vi "ScriptCreateEIO.vi"(8 "direction":T9, 9 "nodes links":string[](array[string]), 10 "Position":cluster{"Left":i32, "Top":i32}, 11 "TopLevelDiagram in":refnum<vi>) -> (0 "terminal names":string[](array[string]), 1 "FPGA I/O out":refnum<vi>, 2 "FPGA I/O in":refnum<vi>, 3 "I/O terminal":refnum<vi>)   [LabVIEW 2014]
uses:
  <vilib>/eio/EIO_TerminalDirection.ctl
  <vilib>/XNodeSupport/XNodeTerm3Array.ctl
  <vilib>/XNodeSupport/XNodeTerm3.ctl
  <vilib>/XNodeSupport/XNodeString.ctl
  <vilib>/XNodeSupport/XNodeVariant.ctl
  <vilib>/XNodeSupport/XNodeRect32.ctl
  <vilib>/XNodeSupport/XNodeInt.ctl
  <vilib>/XNodeSupport/XNodeBool.ctl
  <vilib>/XNodeSupport/XNodeTermDirection.ctl
  <vilib>/eio/EIONode/EIONode.ctl
  <vilib>/eio/XNode/Errors/EIOXNodeErrorStruct.ctl
  <vilib>/eio/XNode/Errors/EIOXNodeInternalErrorTypes.ctl
  <vilib>/eio/XNode/Errors/EIOXNodeUserErrorTypes.ctl
  <vilib>/eio/EIONode/EIONodeElement.ctl
  <vilib>/eio/EIONode/EIONode.xnode
  <vilib>/XNodeSupport/NI_XNodeSupport.lvlib
panel:
  out "terms":T1
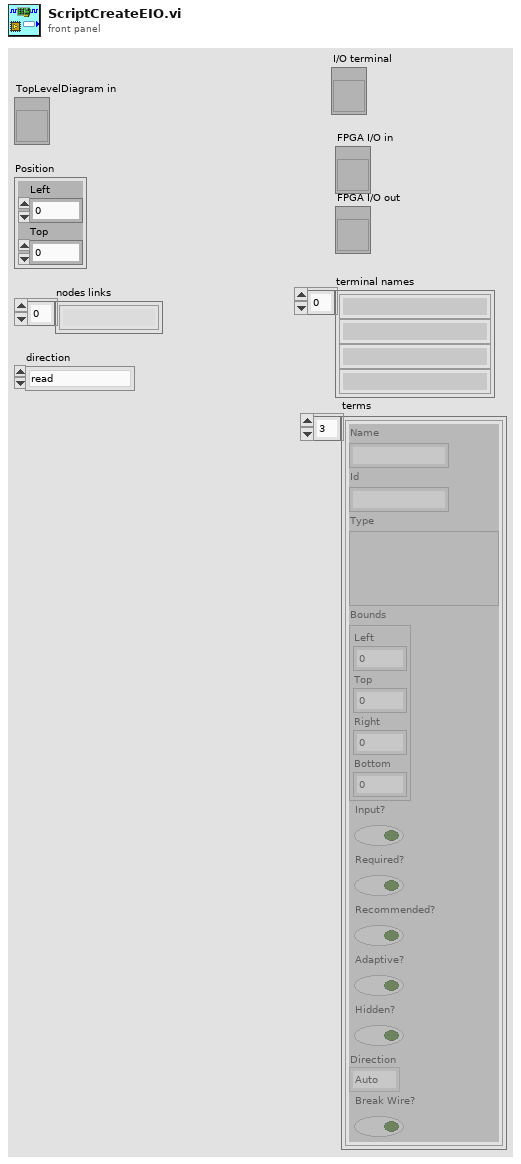
[diagram p1: front panel]
types:
  T1 = typedef "NI_XNodeSupport.lvlib/XNodeTerm3Array.ctl" = T2[]
  T2 = typedef "NI_XNodeSupport.lvlib/XNodeTerm3.ctl" = cluster{"Name":T3, "Id":T3, "Type":T4, "Bounds":T5, "Input?":T7, "Required?":T7, "Recommended?":T7, "Adaptive?":T7, "Hidden?":T7, "Direction":T8, "Break Wire?":T7}
  T3 = typedef "NI_XNodeSupport.lvlib/XNodeString.ctl" = string
  T4 = typedef "NI_XNodeSupport.lvlib/XNodeVariant.ctl" = variant
  T5 = typedef "NI_XNodeSupport.lvlib/XNodeRect32.ctl" = cluster{"Left":T6, "Top":T6, "Right":T6, "Bottom":T6}
  T6 = typedef "NI_XNodeSupport.lvlib/XNodeInt.ctl" = i32
  T7 = typedef "NI_XNodeSupport.lvlib/XNodeBool.ctl" = bool
  T8 = typedef "NI_XNodeSupport.lvlib/XNodeTermDirection.ctl" = enum32{"Auto", "Up", "Down", "Left", "Right", "Center"}
  T9 = typedef "EIO_TerminalDirection.ctl" = enum16{"read", "write", "none", "both"}
  T10 = typedef "EIONodeElement.ctl" = cluster{"alias":string, "direction":T9, "terminal id":string, "type":variant, "wiredtype":variant, "confighash":string, "ref in wired":bool, "ref in type":variant, "uninitialized":bool, "node config":cluster{"name":string, "value":string}[], "id":u32, "generate DFIR?":bool}
  T11 = typedef "EIONode.xnode/EIONode.ctl" = cluster{"error terms":bool, "id counter":u32, "error status":T12, "links":cluster{"alias name":string, "linkage name":string}[], "suppress signature change":bool, "DoSpecify":bool, "elements":T10[], "ignore ref inputs":bool}
  T12 = typedef "EIOXNodeErrorStruct.ctl" = cluster{"internal error list":cluster{"type":T13, "error (no error)":errorcluster}[], "user error list":cluster{"type":T14, "short errors":variant[]}[]}
  T13 = typedef "EIOXNodeInternalErrorTypes.ctl" = enum16{"code generation", "code modification", "node specification", "script plugin", "specify plugin", "config plugin", "script plugin call", "specify plugin call", "config plugin call", "mutation"}
  T14 = typedef "EIOXNodeUserErrorTypes.ctl" = enum16{"code generation", "node specification", "node config"}
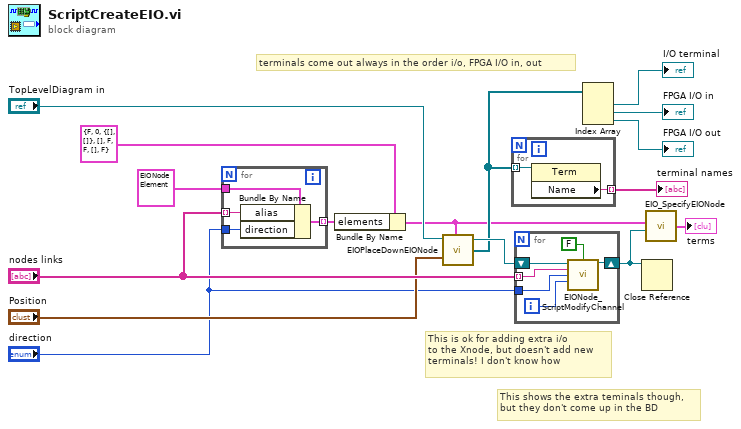
[diagram p0: block diagram]
diagram:
  # "This shows the extra teminals though,\nbut they don't come up in the BD"
  # "This is ok for adding extra i/o\nto the Xnode, but doesn't add new\nterminals! I don't know how"
  # "terminals come out always in the order i/o, FPGA I/O in, out"
  n1 = for {
    tunnel: "nodes links" -> [w20] mode=indexing
    tunnel: [w19] -> w16 mode=indexing
    tunnel: T10 {"alias"="", "direction"=enum."read", "terminal id"="", "type"=variant, "wiredtype"=variant, "confighash"="", "ref in wired"=FALSE, "ref in type"=variant, "uninitialized"=FALSE, "node config"=[], "id"=0, "generate DFIR?"=FALSE} ("element") -> [w18]
    tunnel: "direction" -> [w17]
    n2 = Bundle By Name(cluster=w18, "alias"=w20, "direction"=w17) -> (w19:T10)
  }
  n3 = Bundle By Name(cluster=T11 {"error terms"=FALSE, "id counter"=0, "error status"={"internal error list"=[], "user error list"=[]}, "links"=[], "suppress signature change"=FALSE, "DoSpecify"=FALSE, "elements"=[], "ignore ref inputs"=FALSE} ("State"), "elements"=w16) -> (w3:T11)
  n4 = call <vilib>:"EIOPlaceDownEIONode.vi"("Diagram"="TopLevelDiagram in", "Position"="Position", "State"=w3) -> ("XNode Refnum"=w14:refnum<vi>, "Terms[]"=w10:refnum<vi>[])  [unwired: 2 in, 1 out]
  n5 = for {
    tunnel: w10 -> [w22] mode=indexing
    tunnel: [w21] -> w9 mode=indexing
    n6 = property class="Term"(reference=w22) -> ("Name"=w21:string)  [unwired: 1 in, 2 out]
  }
  "terminal names" <- w9
  n7 = for {
    shift-right: [w25] -> w2
    shift-left: w14 -> [w28]
    tunnel: "nodes links" -> [w27] mode=indexing
    tunnel: "direction" -> [w26]
    i -> [w24]
    n8 = call <vilib>:"EIONode_ScriptModifyChannel.vi"("node"=w28, "error terms"=FALSE, "name"=w27, "direction"=w26, "index"=w24) -> ("node out"=w25:refnum<vi>)  [unwired: 9 in, 1 out]
  }
  n9 = Index Array(array=w10) -> (element #1=→"I/O terminal":refnum<vi>, element #2=→"FPGA I/O in":refnum<vi>, element #3=→"FPGA I/O out":refnum<vi>)  [unwired: 3 in]
  n10 = Close Reference(reference=w2) -> ()  [unwired: 1 in, 1 out]
  n11 = call <vilib>:"EIO_SpecifyEIONode.vi"("node/diagram"=w2, "State In"=w3) -> ("terms"=→"terms":T1)  [unwired: 2 in]
